vi "Configure Batch.vi"(0 "VISA resource name":refnum<visa-resource-name>, 5 "Enable Batch Function (Disable)":bool, 7 "Lot-No. Digit (6)":u16(ring)=6 items=["Off"=0, "4"=4, "6"=6, "8"=8], 9 "Auto Increment (ON)":bool=TRUE, 11 "error in (no error)":errorcluster) -> (4 "VISA resource name out":refnum<visa-resource-name>, 15 "error out":errorcluster)   [LabVIEW 2020, in "Yokogawa GX Series.lvlib"]
doc: "Sets the batch function.\n\nCommand: SBatch"
uses:
  <instrlib>/Yokogawa GX Series/Yokogawa GX Series.lvlib
panel:
  in  "Recording start display":i32(ring)=1 items=["Batch Comment", "Text Field"]
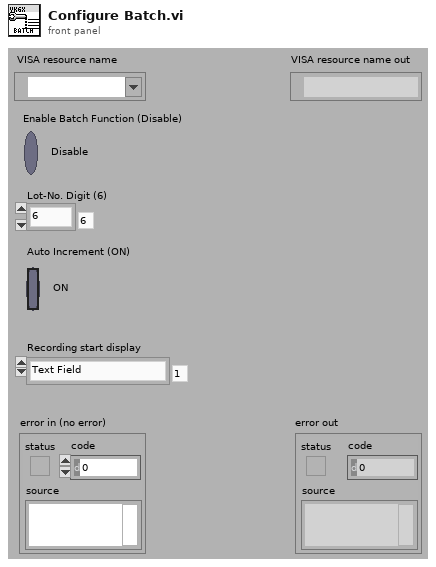
[diagram p1: front panel]
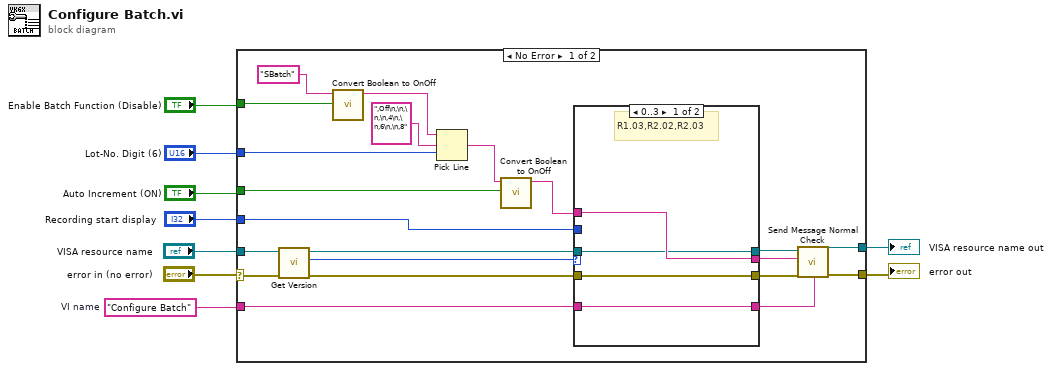
[diagram p0: block diagram]
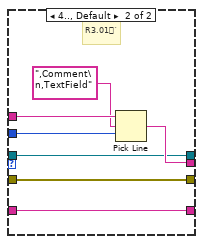
[diagram p2: hidden frame]
diagram:
  w8 = "Configure Batch"  # VI name
  n1 = case shown="No Error" "error in (no error)" {
    selector: "error in (no error)" -> [w20 w42]
    tunnel: "VISA resource name" -> [w21 w43]
    tunnel: w8 -> [w12 _]
    tunnel: [w30 w43] -> w7
    tunnel: [w29 w42] -> w6
    tunnel: "Lot-No. Digit (6)" -> [w27 _]
    tunnel: "Enable Batch Function (Disable)" -> [w25 _]
    tunnel: "Auto Increment (ON)" -> [w22 _]
    tunnel: "Recording start display" -> [w10 _]
    frame No Error {
      n2 = call <instrlib>:"Get Version.vi"("error in (no error)"=w20, "VISA resource name"=w21) -> ("error out"=w14:errorcluster, "Version"=w19:i32, "VISA resource name out"=w16:refnum<visa-resource-name>)  [unwired: 7 in]
      n3 = call <instrlib>:"Convert Boolean to OnOff.vi"("On/Off"=w25, "Initial String (\"\")"="SBatch") -> ("Resulting String"=w24:string)  [unwired: 9 in]
      n4 = Pick Line(string ("")=w24, multi-line string=",Off\n,\n,\n,\n,4\n,\n,6\n,\n,8", line index=w27) -> (output string=w23:string)
      n5 = call <instrlib>:"Convert Boolean to OnOff.vi"("On/Off"=w22, "Initial String (\"\")"=w23) -> ("Resulting String"=w18:string)  [unwired: 9 in]
      n6 = case shown="0..3" w19 {
        tunnel: w18 -> [w34 w41]
        tunnel: [w34 w38] -> w17
        tunnel: w16 -> [w33 w37]
        tunnel: [w33 w37] -> w15
        tunnel: w14 -> [w32 w36]
        tunnel: [w32 w36] -> w13
        tunnel: w12 -> [w31 w35]
        tunnel: [w31 w35] -> w11
        tunnel: w10 -> [_ w40]
        frame 0..3 {
          # "R1.03,R2.02,R2.03"
        }
        frame 4.., Default {
          # "R3.01`"
          n7 = Pick Line(string ("")=w41, multi-line string=",Comment\n,TextField", line index=w40) -> (output string=w38:string)
        }
      }
      n8 = call <instrlib>:"Send Message Normal Check.vi"("Source (\"\")"=w11, "error in (no error)"=w13, "Send Message (\"\")"=w17, "VISA resource name"=w15) -> ("error out"=w29:errorcluster, "VISA resource name out"=w30:refnum<visa-resource-name>)  [unwired: 2 in, 4 out]
    }
    frame Error {
    }
  }
  "error out" <- w6
  "VISA resource name out" <- w7
